vi "Parse All Notes.vi"(8 "error in (no error)":errorcluster, 10 "SR Cluster in":T1 {"Creation Date" format="%<%x>T"; "Last Updated" format="%<%x>T"}, 11 "result string":string) -> (0 "error out":errorcluster, 2 "SR Cluster out":T1 {"Creation Date" format="%<%x>T"; "Last Updated" format="%<%x>T"}, 3 "Array":T3[](array[typedef]) {"Note Date" format="%<%x >T"})   [LabVIEW 2018]
uses:
  Type Defs/SR Note Cluster.ctl
  Type Defs/SR Cluster.ctl
  Type Defs/SR Status.ctl
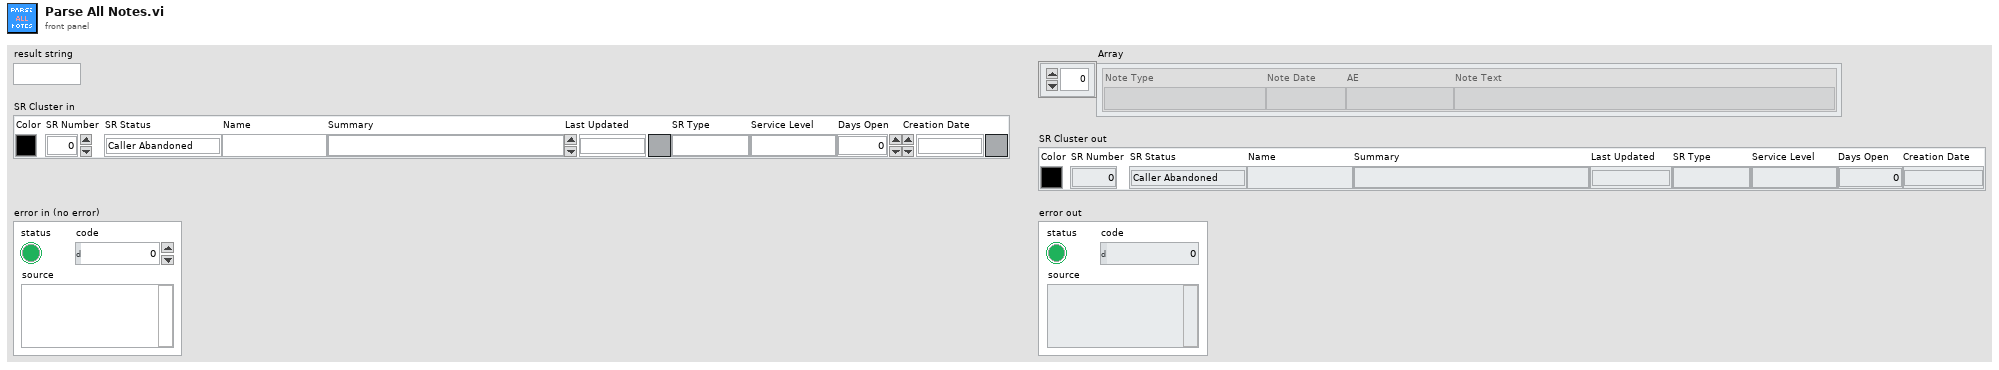
[diagram p1: front panel]
types:
  T1 = typedef "SR Cluster.ctl" = cluster{"Color":u32, "SR Number":i32, "SR Status":T2, "Name":string, "Summary":string, "Last Updated":timestamp, "SR Type":string, "Service Level":string, "Days Open":dbl, "Creation Date":timestamp}
  T2 = typedef "SR Status.ctl" = enum16{"Caller Abandoned", "Created in Error", "Expired", "Forum Resolved AE", "Forum Resolved Customer", "IN WORK", "IN WORK Collab with AES", "IN WORK Collab with PSE", "IN WORK Collab with SE", "IN WORK Customer Added Note", "IN WORK Escalation", "IN WORK Wait on Customer", "Open", "Potentially Resolved", "Presumed Resolved", "RMA Approved for Return", "Resolved", "Passed Off"}
  T3 = typedef "SR Note Cluster.ctl" = cluster{"Note Type":string, "Note Date":timestamp, "AE":string, "Note Text":string}
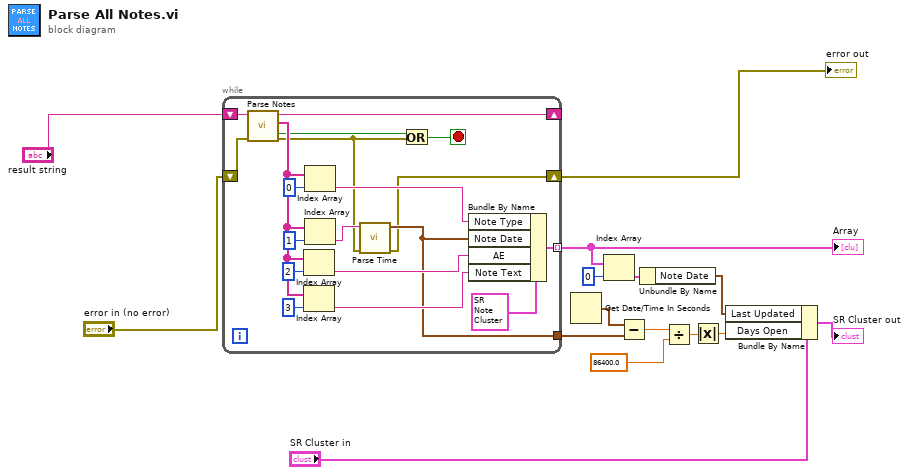
[diagram p0: block diagram]
diagram:
  n1 = while {
    shift-right: [w33] -> _
    shift-left: "result string" -> [w34]
    tunnel: [w22] -> w3 mode=indexing
    tunnel: [w18] -> w8
    shift-right: [w17] -> w14
    shift-left: "error in (no error)" -> [w32]
    stop <- w21 stop-if-true
    n2 = call "Parse Notes.vi"("error in"=w32, "String"=w34) -> ("error out"=w16:errorcluster, "Done Reading?"=w20:bool, "sr note out"=w31:string[], "result string out"=w33:string)  [unwired: 6 in]
    n3 = Index Array(array=w31, index=2) -> (element=w24:string)
    n4 = Index Array(array=w31, index=3) -> (element=w25:string)
    n5 = Index Array(array=w31, index=0) -> (element=w23:string)
    n6 = Index Array(array=w31, index=1) -> (element=w19:string)
    n7 = call "Parse Time.vi"("error in (no error)"=w16, "data"=w19) -> ("error out"=w17:errorcluster, "Time Stamp"=w18:timestamp)  [unwired: 8 in]
    n8 = Or(x=w20, y=w16) -> (x .or. y?=w21:bool)
    n9 = Bundle By Name(cluster=T3 {"Note Type"="", "Note Date"=timestamp(0 s since 1904-01-01), "AE"="", "Note Text"=""} ("SR Note Cluster"), "Note Type"=w23, "Note Date"=w18, "AE"=w24, "Note Text"=w25) -> (w22:T3)
  }
  "error out" <- w14
  "Array" <- w3
  n10 = Get Date/Time In Seconds() -> (seconds since 1Jan1904=w7:timestamp)
  n11 = Index Array(array=w3, index=0) -> (element=w5:T3)
  n12 = Subtract(x=w7, y=w8) -> (x-y=w9:dbl)
  n13 = Unbundle By Name(w5) -> ("Note Date"=w6:timestamp)
  n14 = Divide(x=w9, y=86400.0) -> (x/y=w12:dbl)
  n15 = Absolute Value(x=w12) -> (abs(x)=w13:dbl)
  n16 = Bundle By Name(cluster="SR Cluster in", "Last Updated"=w6, "Days Open"=w13) -> (→"SR Cluster out":T1)
